vi "Tacking Helper - Wind Plot.vi"(9 "Boat\nPosition":T2, 10 "Wind Vector\nTop = x\nBottom = y":T1, 11 "Wind Vector\nScaling Factor":dbl) -> (3 "Output Cluster\nFor Plotting":cluster{dbl[], dbl[]})   [LabVIEW 2011]
doc: "This packages the wind vector into a form appropriate for plotting in the front panel - separate arrays of x and y data clustered together. The wind vector is also scaleable so it can be seen easily"
uses:
  2 Typedefs/UTM Location.ctl
  2 Typedefs/Velocity.ctl
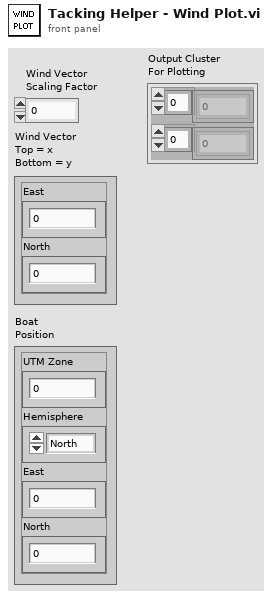
[diagram p1: front panel]
types:
  T1 = typedef "Velocity.ctl" = cluster{"East":dbl, "North":dbl}
  T2 = typedef "UTM Location.ctl" = cluster{"UTM Zone":dbl, "Hemisphere":enum16{"North", "South"}, "East":dbl, "North":dbl}
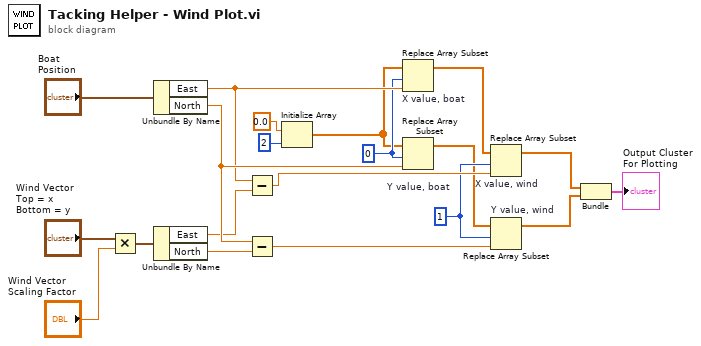
[diagram p0: block diagram]
diagram:
  w9 = 0 ("index")
  w10 = 1 ("index")
  n1 = Multiply(x="Wind Vector\nTop = x\nBottom = y", y="Wind Vector\nScaling Factor") -> (x*y=w18:T1)
  n2 = Unbundle By Name("Boat\nPosition") -> ("East"=w13:dbl, "North"=w15:dbl)
  n3 = Unbundle By Name(w18) -> ("East"=w12:dbl, "North"=w14:dbl)
  n4 = Subtract(x=w13, y=w12) -> (x-y=w11:dbl)
  n5 = Subtract(x=w15, y=w14) -> (x-y=w17:dbl)
  n6 = Initialize Array "Initialize Array"(0.0 ("element"), 2 ("dimension size")) -> (w5:dbl[])
  n7 = Replace Array Subset "X value, boat"(array=w5, new element=w13, index=w9) -> (w3:dbl[])
  n8 = Replace Array Subset "Y value, boat"(array=w5, new element=w15, index=w9) -> (w4:dbl[])
  n9 = Replace Array Subset "X value, wind"(array=w3, new element=w11, index=w10) -> (w6:dbl[])
  n10 = Replace Array Subset "Y value, wind"(array=w4, new element=w17, index=w10) -> (w7:dbl[])
  n11 = Bundle(w6, w7) -> (→"Output Cluster\nFor Plotting":cluster{dbl[], dbl[]})  [unwired: 1 in]
